vi "Example Authenticate - EnumerateCallback Callback.vi"(4 "EnumerateCallback":refnum<user-event>, 5 "Event Data":T1, 6 "Control Ref":refnum<k24>, 7 "Event Common Data":T2) -> ()   [LabVIEW 2010]
uses:
  C:/tf/play/labview/Tinkerforge.dll
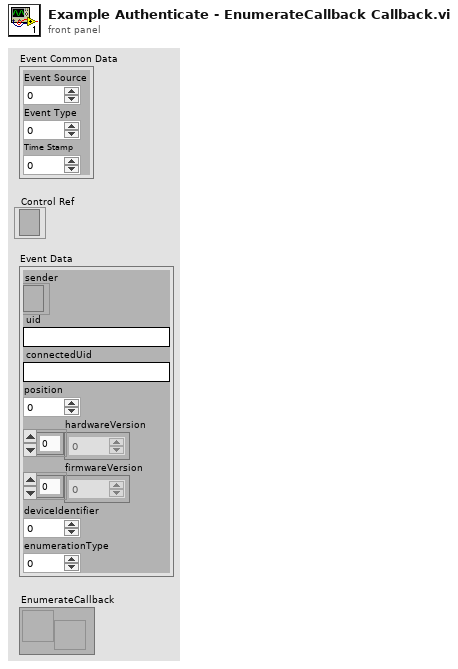
[diagram p1: front panel]
types:
  T1 = cluster{"sender":refnum<k24>, "uid":string, "connectedUid":string, "position":u16, "hardwareVersion":i16[], "firmwareVersion":i16[], "deviceIdentifier":i32, "enumerationType":i16}
  T2 = cluster{"Event Source":i32, "Event Type":u32, "Time Stamp":u32}
  T3 = cluster{"uid":string, "connectedUid":string, "position":u16, "hardwareVersion":i16[], "firmwareVersion":i16[], "deviceIdentifier":i32, "enumerationType":i16}
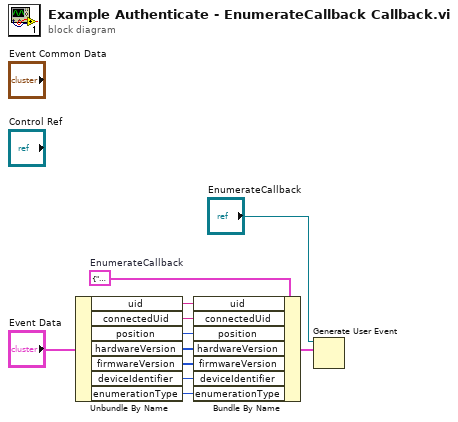
[diagram p0: block diagram]
diagram:
  w10 = T3 {"uid"="", "connectedUid"="", "position"=0, "hardwareVersion"=[], "firmwareVersion"=[], "deviceIdentifier"=0, "enumerationType"=0}  # EnumerateCallback
  n1 = Unbundle By Name("Event Data") -> ("uid"=w9:string, "connectedUid"=w8:string, "position"=w7:u16, "hardwareVersion"=w6:i16[], "firmwareVersion"=w5:i16[], "deviceIdentifier"=w4:i32, "enumerationType"=w3:i16)
  n2 = Bundle By Name(cluster=w10, "uid"=w9, "connectedUid"=w8, "position"=w7, "hardwareVersion"=w6, "firmwareVersion"=w5, "deviceIdentifier"=w4, "enumerationType"=w3) -> (w2:T3)
  n3 = Generate User Event(user event="EnumerateCallback", event data cluster=w2) -> ()  [unwired: 1 in, 2 out]
